vi "Timer.vi"(7 "Method":T1(ring)=enum."Get Elapsed Time", 8 "error in (no error)":errorcluster, 10 "Timeout":dbl, 11 "BehaviorData in":refnum<class "BehaviorData.lvclass">) -> (0 "error out":errorcluster, 1 "Timeout":bool, 2 "Time":dbl, 3 "BehaviorData out":refnum<class "BehaviorData.lvclass">)   [LabVIEW 2010, in "BehaviorData.lvclass"]
uses:
  BehaviorData.lvclass
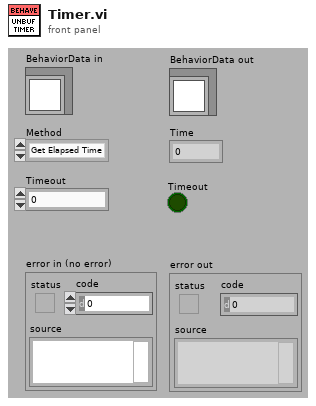
[diagram p1: front panel]
types:
  T1 = enum16{"Get Time", "Get Elapsed Time", "Reset Elapsed Time"}
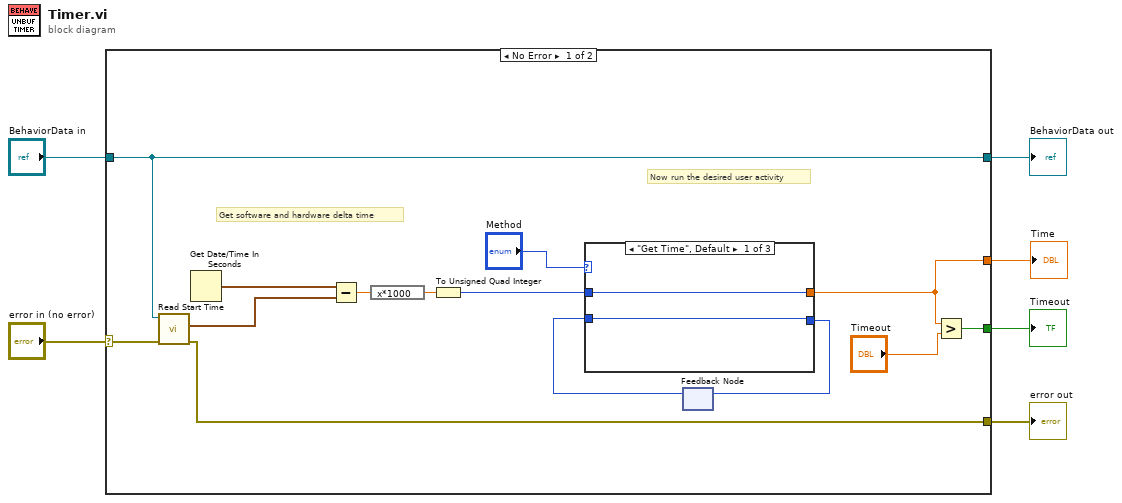
[diagram p0: block diagram]
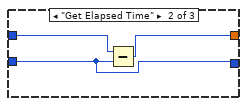
[diagram p2: hidden frame]
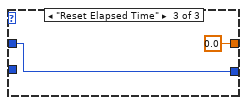
[diagram p3: hidden frame]
diagram:
  n1 = case shown="No Error" "error in (no error)" {
    selector: "error in (no error)" -> [w8 w29]
    tunnel: [w7 w29] -> w5
    tunnel: [w10 w28] -> w3
    tunnel: "BehaviorData in" -> [w10 w28]
    tunnel: [w14 _] -> w2
    tunnel: [w12 _] -> w1
    frame No Error {
      # "Now run the desired user activity"
      # "Get software and hardware delta time"
      n2 = call-dynamic "Read Start Time.vi"("error in (no error)"=w8, "AcquistionObject in"=w10) -> ("error out"=w7:errorcluster, "Start Time"=w9:timestamp)  [unwired: 7 in, 1 out]
      n3 = Get Date/Time In Seconds() -> (seconds since 1Jan1904=w20:timestamp)
      n4 = Subtract(x=w20, y=w9) -> (x-y=w19:dbl)
      n5 = expression code="x*1000"(w19) -> (w18:dbl)
      n6 = To Unsigned Quad Integer(1:w18) -> (0:w11:u64)
      n7 = feedback #1() -> (w16:u64)  [unwired: 1 in]
      n8 = case shown="\"Get Time\", Default" "Method" {
        tunnel: w11 -> [w22 w25 w27]
        tunnel: [w22 w24 0.0] -> w14
        tunnel: w16 -> [w21 w23 _]
        tunnel: [w21 w23 w27] -> w15
        frame "Get Time", Default {
        }
        frame "Get Elapsed Time" {
          n9 = Subtract(x=w25, y=w23) -> (x-y=w24:u64)
        }
        frame "Reset Elapsed Time" {
        }
      }
      n10 = feedback-in #1(w15) -> ()
      n11 = Greater?(x=w14, y="Timeout") -> (0:w12:bool)
    }
    frame Error {
    }
  }
  "error out" <- w5
  "BehaviorData out" <- w3
  "Time" <- w2
  "Timeout" <- w1
